vi "Visa Read and Write 2 .vi"() -> ()   [LabVIEW 2016]
uses:
  <vilib>/Instr/_visa.llb/VISA Configure Serial Port (Instr).vi
panel:
  out "decimal integer string":string
  out "led":bool
  out "Gauge":dbl(knob) scale=0.0..5.0
  in  "stop":bool
  in  "VISA resource name":refnum<visa-resource-name>
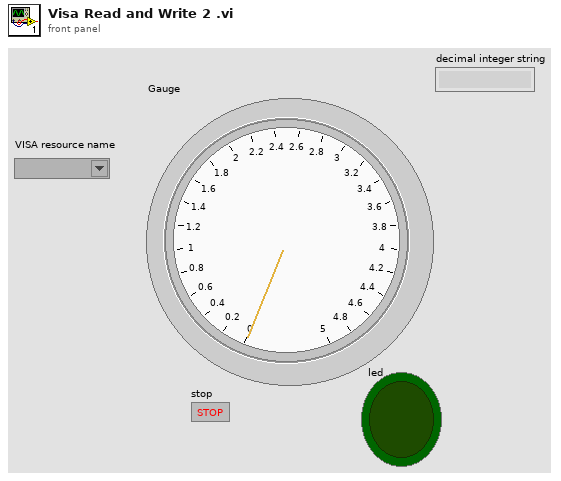
[diagram p1: front panel]
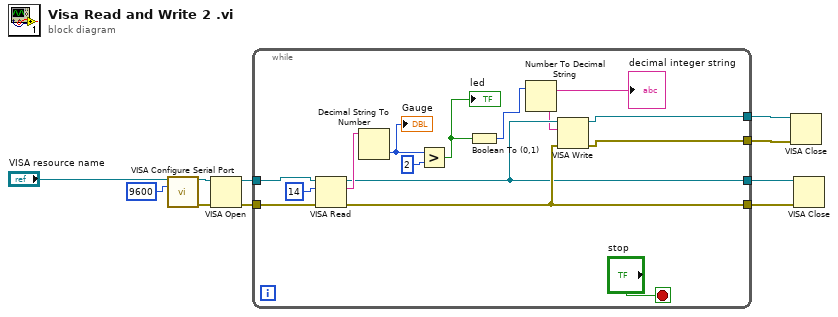
[diagram p0: block diagram]
diagram:
  n1 = call-poly "VISA Configure Serial Port"("VISA resource name"="VISA resource name", "baud rate (9600)"=u32 9600) -> ("VISA resource name out"=w9:refnum<visa-resource-name>, "error out"=w10:errorcluster)  [unwired: 12 in]
  n2 = VISA Open(error in (no error)=w10, VISA resource name=w9) -> (VISA resource name=w8:refnum<visa-resource-name>, error out=w7:errorcluster)  [unwired: 3 in]
  n3 = while {
    tunnel: w8 -> [w24]
    tunnel: w7 -> [w23]
    tunnel: [w17] -> w6
    tunnel: [w16] -> w5
    tunnel: [w15] -> w2
    tunnel: [w14] -> w1
    stop <- "stop" stop-if-true
    n4 = VISA Read(VISA resource name=w24, byte count=u32 14, error in (no error)=w23) -> (VISA resource name out=w16:refnum<visa-resource-name>, read buffer=w22:string, error out=w17:errorcluster)  [unwired: 1 out]
    n5 = Decimal String To Number(string=w22) -> (number=w19:i32)  [unwired: 2 in, 1 out]
    "Gauge" <- w19
    n6 = Greater?(x=w19, y=2 ("x")) -> (0:w13:bool)
    "led" <- w13
    n7 = Boolean To (0,1)(Boolean=w13) -> (0, 1=w12:i16)
    n8 = Number To Decimal String(number=w12) -> (decimal integer string=w11:string)  [unwired: 1 in]
    "decimal integer string" <- w11
    n9 = VISA Write(VISA resource name=w16, write buffer=w11, error in (no error)=w17) -> (VISA resource name out=w15:refnum<visa-resource-name>, error out=w14:errorcluster)  [unwired: 1 out]
  }
  n10 = VISA Close(VISA resource name=w2, error in (no error)=w1) -> ()  [unwired: 1 out]
  n11 = VISA Close(VISA resource name=w5, error in (no error)=w6) -> ()  [unwired: 1 out]
